vi "createSineWave.vi"(4 "phase":dbl, 6 "sampleRate":dbl, 7 "duration":dbl, 8 "error in (no error)":errorcluster, 9 "Amplitude":dbl, 10 "freq":dbl, 11 "SoundDeviceData in":refnum<class "SoundDeviceData.lvclass">) -> (0 "error out":errorcluster, 1 "phase out":dbl format="%^#_6g", 2 "sineWave":dbl[](array[numeric]), 3 "SoundDeviceData out":refnum<class "SoundDeviceData.lvclass">)   [LabVIEW 2009, in "DataMappers.lvlib" / "SoundDeviceData.lvclass"]
uses:
  SoundDeviceData.lvclass
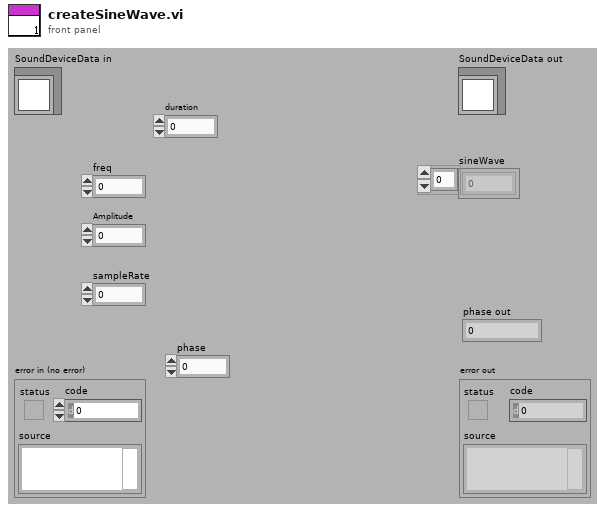
[diagram p1: front panel]
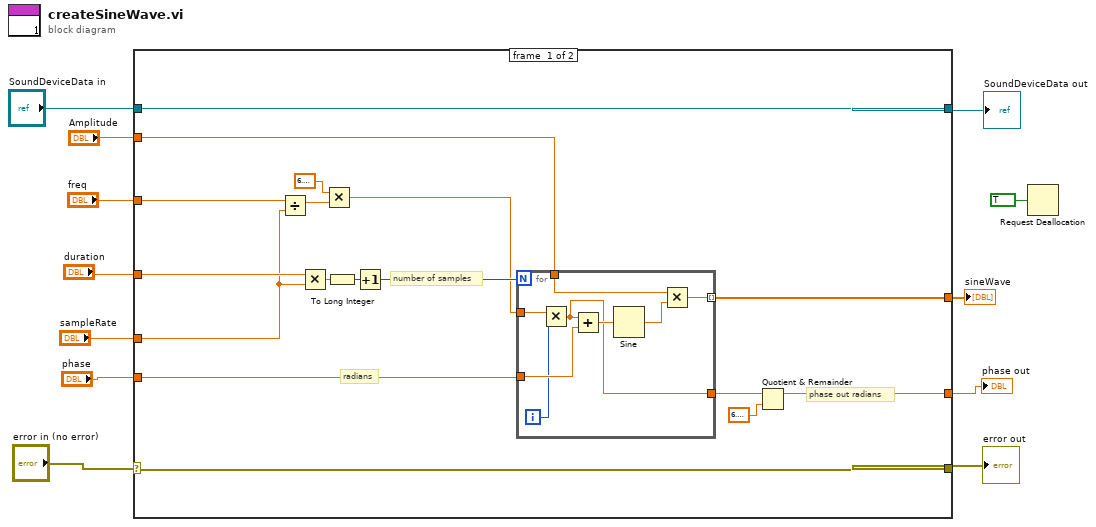
[diagram p0: block diagram]
diagram:
  n1 = case shown="No Error" "error in (no error)" {
    selector: "error in (no error)" -> [w28 w39]
    tunnel: [w28 w39] -> w11
    tunnel: [w29 w38] -> w9
    tunnel: "SoundDeviceData in" -> [w29 w38]
    tunnel: "Amplitude" -> [w19 _]
    tunnel: "freq" -> [w18 _]
    tunnel: "duration" -> [w17 _]
    tunnel: "sampleRate" -> [w16 _]
    tunnel: "phase" -> [w15 _]
    tunnel: [w14 _] -> w3
    tunnel: [w13 _] -> w2
    frame #0 {
      # "radians"
      # "phase out radians"
      # "number of samples"
      n2 = Divide(x=w18, y=w16) -> (x/y=w26:dbl)
      n3 = Multiply(x=w17, y=w16) -> (x*y=w22:dbl)
      n4 = Multiply(x=6.283185307179586, y=w26) -> (x*y=w23:dbl)
      n5 = To Long Integer(number=w22) -> (32bit integer=w25:i32)
      n6 = Increment(x=w25) -> (x+1=w24:i32)
      n7 = for {
        N: w24 -> [_]
        tunnel: w19 -> [w37]
        tunnel: [w35] -> w13 mode=indexing
        tunnel: w15 -> [w33]
        tunnel: w23 -> [w32]
        tunnel: [w30] -> w20
        i -> [w31]
        n8 = Multiply(x=w32, y=w31) -> (x*y=w30:dbl)
        n9 = Add(x=w30, y=w33) -> (x+y=w34:dbl)
        n10 = Sine(x=w34) -> (sin(x)=w36:dbl)
        n11 = Multiply(x=w37, y=w36) -> (x*y=w35:dbl)
      }
      n12 = Quotient & Remainder(x=w20, y=6.283185307179586) -> (x-y*floor(x/y)=w14:dbl)  [unwired: 1 out]
    }
    frame #1 {
    }
  }
  "error out" <- w11
  "SoundDeviceData out" <- w9
  "phase out" <- w3
  "sineWave" <- w2
  n13 = Request Deallocation(TRUE) -> ()
